vi "Buffer Connections List_Actions.vi"(0 "Connection Cluster":T2, 1 "ref in":T3, 2 "State":T1=enum."Update", 7 "index":i32, 11 "error in (no error)":errorcluster) -> (3 "ref out":T3, 4 "Connections":T2[](array[typedef]), 8 "Connection Cluster Out":T2, 15 "error out":errorcluster {"code" min=0 max=0})   [LabVIEW 2013, in "J1939.lvlib"]
uses:
  J1939.lvlib
  BAM/BAM Buffer Connections List_Ref.ctl
  TP/TP Buffer Connection Cluster.ctl
  TP/TP Connections List State.ctl
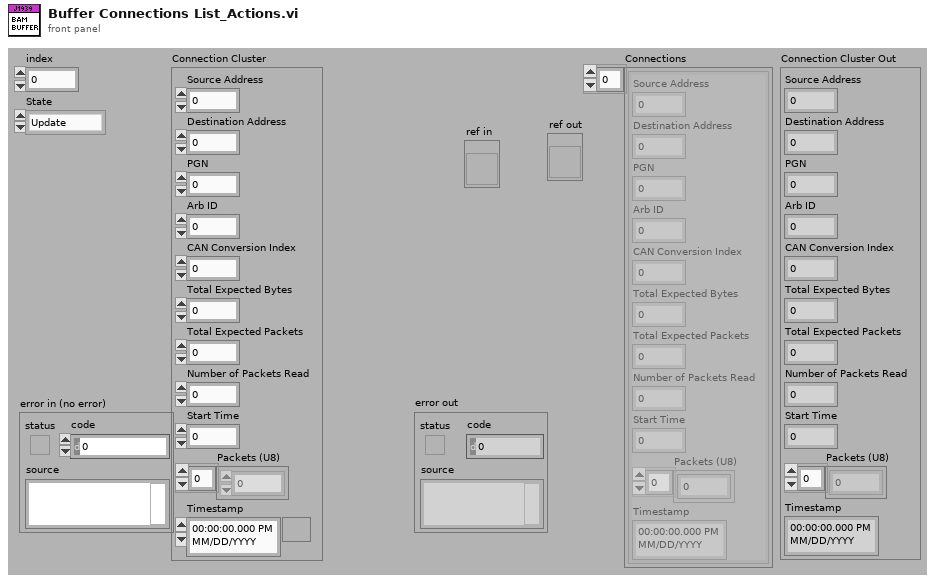
[diagram p1: front panel]
types:
  T1 = typedef "J1939.lvlib/TP Connections List State.ctl" = enum16{"Add", "Update", "Get", "Remove", "Initialize"}
  T2 = typedef "J1939.lvlib/TP Buffer Connection Cluster.ctl" = cluster{"Source Address":u8, "Destination Address":u8, "PGN":u32, "Arb ID":u32, "CAN Conversion Index":u32, "Total Expected Bytes":u16, "Total Expected Packets":u8, "Number of Packets Read":u8, "Start Time":u32, "Packets (U8)":u8[], "Timestamp":timestamp}
  T3 = typedef "J1939.lvlib/BAM Buffer Connections List_Ref.ctl" = refnum<vi>
  T4 = typedef "J1939 TP Buffer Connection Cluster.ctl" = cluster{"Source Address":u8, "Destination Address":u8, "PGN":u32, "Arb ID":u32, "CAN Conversion Index":u32, "Total Expected Bytes":u16, "Total Expected Packets":u8, "Number of Packets Read":u8, "Start Time":u32, "Packets (U8)":u8[], "Timestamp":timestamp}
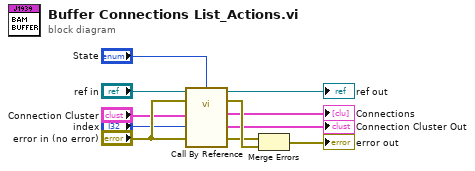
[diagram p0: block diagram]
diagram:
  n1 = call-by-ref "?"(reference="ref in", error in="error in (no error)", "Connection Cluster"="Connection Cluster", "State"="State", "index"="index", 11:"error in (no error)"="error in (no error)") -> (reference out=→"ref out":T3, error out=w10:errorcluster, "Connections"=→"Connections":T4[], "Connection Cluster Out"=→"Connection Cluster Out":T4, 15:"error out"=w9:errorcluster)  [unwired: 9 in]
  n2 = Merge Errors(w9, w10) -> (→"error out":errorcluster)
